vi "VI Server_TREE_ColumnHeader_Names_SET.vi"(6 "Column Header Strings[]":string[](array[string]), 7 "Label":string, 8 "error in":errorcluster, 9 "Tree.Ref":refnum<vi>, 11 "VI Server.RefsCluster":T1) -> (0 "error out":errorcluster, 1 "Tree.Ref.DUP":refnum<vi>, 3 "VI Server.RefsCluster.DUP":T1)   [LabVIEW 2020]
uses:
  VI Server_TypeDefs/VI Server_RefsCluster.ctl
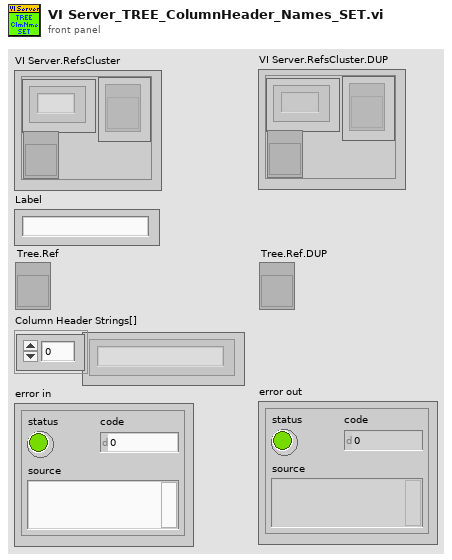
[diagram p1: front panel]
types:
  T1 = typedef "VI Server_RefsCluster.ctl" = cluster{"Labels":string[], "Refs":refnum<vi>[], "VI Ref":refnum<vi>}
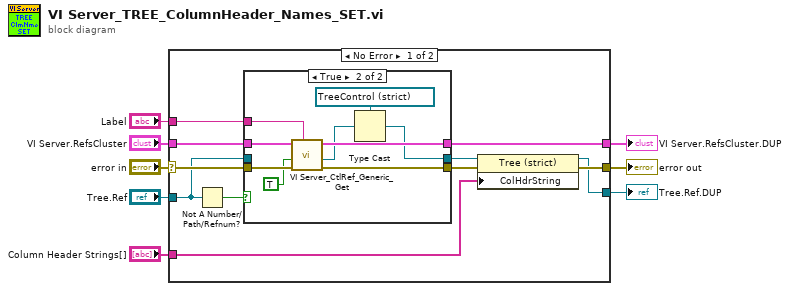
[diagram p0: block diagram]
diagram:
  n1 = case shown="No Error" "error in" {
    selector: "error in" -> [w19 w33]
    tunnel: [w13 w33] -> w7
    tunnel: "VI Server.RefsCluster" -> [w18 w32]
    tunnel: [w17 w32] -> w5
    tunnel: "Label" -> [w16 _]
    tunnel: [w12 _] -> w1
    tunnel: "Column Header Strings[]" -> [w11 _]
    tunnel: "Tree.Ref" -> [w9 _]
    frame No Error {
      n2 = Not A Number/Path/Refnum?(number/path/refnum=w9) -> (NaN/Path/Refnum?=w10:bool)
      n3 = case shown="True" w10 {
        tunnel: w19 -> [w22 w31]
        tunnel: w18 -> [w21 w30]
        tunnel: [w21 w29] -> w17
        tunnel: w16 -> [_ w28]
        tunnel: [w22 w26] -> w15
        tunnel: [w20 w25] -> w14
        tunnel: w9 -> [w20 _]
        frame False {
        }
        frame True {
          n4 = call "VI Server_CtlRef_Generic_Get.vi"("Control.Label"=w28, "error in"=w31, "SingleInstance"=TRUE, "VI Server.RefsCluster"=w30) -> ("error out"=w26:errorcluster, "Control.Ref.Generic"=w27:refnum<vi>, "VI Server.RefsCluster.DUP"=w29:T1)  [unwired: 5 in]
          n5 = Type Cast(type=refnum<vi> refnum ("Test.Tree"), x=w27) -> (*(type *) &x=w25:refnum<vi>)
        }
      }
      n6 = property class="Tree (strict)"(reference=w14, error in=w15, "ColHdrString"=w11) -> (reference out=w12:refnum<vi>, error out=w13:errorcluster)
    }
    frame Error {
    }
  }
  "VI Server.RefsCluster.DUP" <- w5
  "error out" <- w7
  "Tree.Ref.DUP" <- w1
